vi "CreateLaserPowerTask.vi"(8 "error in":errorcluster) -> (0 "error out":errorcluster, 3 "task out":refnum<k21>)   [LabVIEW 2015]
uses:
  <vilib>/DAQmx/create/channels.llb/DAQmx Create Channel (AO-Voltage-Basic).vi
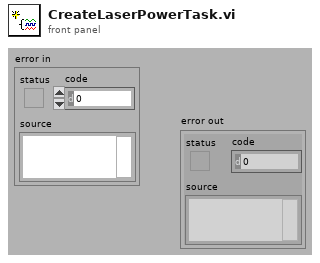
[diagram p1: front panel]
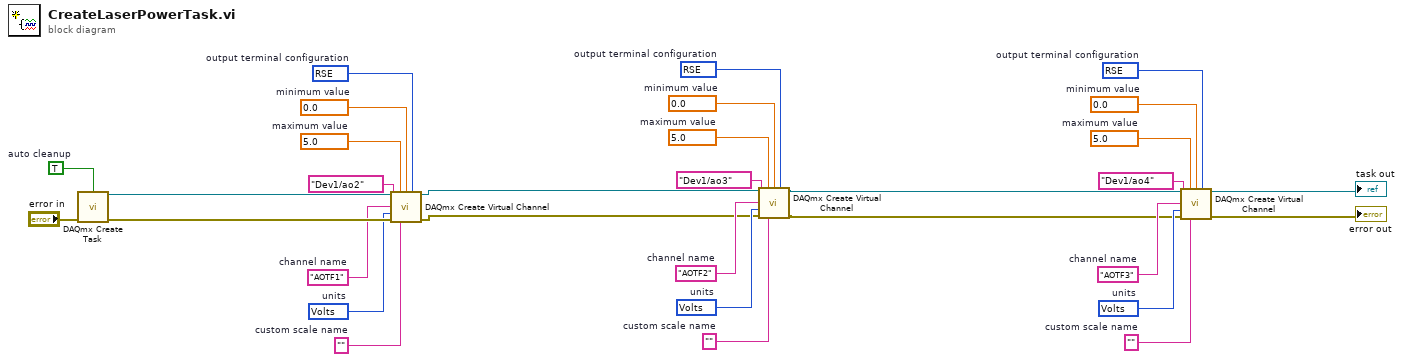
[diagram p0: block diagram]
diagram:
  w10 = 10083 items=["Default"=-1, "RSE"=10083, "Differential"=10106, "Pseudodifferential"=12529]  # output terminal configuration
  w11 = 10348 items=["Volts"=10348, "From Custom Scale"=10065]  # units
  w12 = "AOTF3"  # channel name
  w13 = ""  # custom scale name
  w14 = 0.0  # minimum value
  w15 = 5.0  # maximum value
  w16 = 10083 items=["Default"=-1, "RSE"=10083, "Differential"=10106, "Pseudodifferential"=12529]  # output terminal configuration
  w17 = 10348 items=["Volts"=10348, "From Custom Scale"=10065]  # units
  w18 = "AOTF2"  # channel name
  w19 = ""  # custom scale name
  w20 = 0.0  # minimum value
  w21 = 5.0  # maximum value
  w22 = 10083 items=["Default"=-1, "RSE"=10083, "Differential"=10106, "Pseudodifferential"=12529]  # output terminal configuration
  w23 = 10348 items=["Volts"=10348, "From Custom Scale"=10065]  # units
  w24 = "AOTF1"  # channel name
  w25 = ""  # custom scale name
  w26 = 0.0  # minimum value
  w27 = 5.0  # maximum value
  w29 = TRUE  # auto cleanup
  n1 = call <vilib>:"DAQmx Create Task.vi"("auto cleanup"=w29, "error in"="error in") -> ("task out"=w28:refnum<k21>, "error out"=w30:errorcluster)  [unwired: 12 in]
  n2 = call-poly <vilib>:"DAQmx Create Virtual Channel.vi"("task in"=w28, "maximum value"=w27, "minimum value"=w26, "output terminal configuration"=w22, "physical channels"=tag "Dev1/ao2", "name to assign"=w24, "units"=w23, "error in"=w30, "custom scale name"=w25) -> ("task out"=w9:refnum<k21>, "error out"=w8:errorcluster)  [unwired: 5 in]
  n3 = call-poly <vilib>:"DAQmx Create Virtual Channel.vi"("task in"=w9, "maximum value"=w21, "minimum value"=w20, "output terminal configuration"=w16, "physical channels"=tag "Dev1/ao3", "name to assign"=w18, "units"=w17, "error in"=w8, "custom scale name"=w19) -> ("task out"=w7:refnum<k21>, "error out"=w6:errorcluster)  [unwired: 5 in]
  n4 = call-poly <vilib>:"DAQmx Create Virtual Channel.vi"("task in"=w7, "maximum value"=w15, "minimum value"=w14, "output terminal configuration"=w10, "physical channels"=tag "Dev1/ao4", "name to assign"=w12, "units"=w11, "error in"=w6, "custom scale name"=w13) -> ("task out"=→"task out":refnum<k21>, "error out"=→"error out":errorcluster)  [unwired: 5 in]
